vi "Start Sync.vi"(8 "error in (no error)":errorcluster, 11 "gRPC Server in":refnum<class "RouteGuide.lvclass">) -> (0 "error out":errorcluster, 3 "gRPC Server out":refnum<class "RouteGuide.lvclass">)   [LabVIEW 2019, in "route_guide_server.lvlib" / "RouteGuide.lvclass"]
uses:
  RouteGuide.lvclass
  RouteGuide.lvclass/RouteGuide.ctl
  RPC Messages/routeguide_Feature.ctl
  RPC Messages/routeguide_Point.ctl
  RPC Messages/routeguide_RouteSummary.ctl
  Is Call Cancelled Global.vi
  Server Error Global.vi
  route_guide_server.lvlib
  <vilib>/gRPC/LabVIEW gRPC Library/grpc-lvsupport-release.lvlib
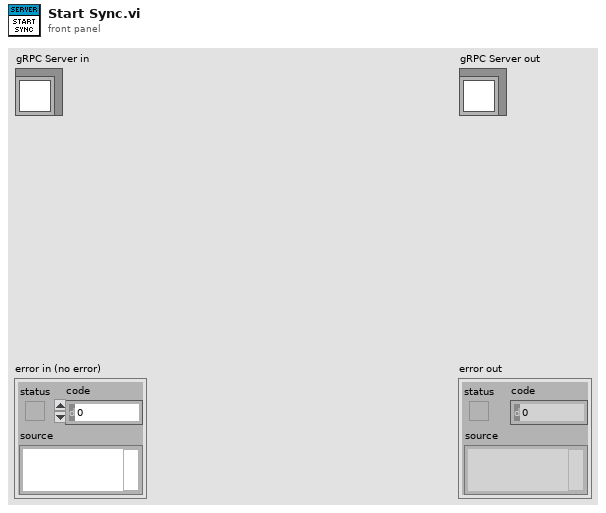
[diagram p1: front panel]
types:
  T1 = typedef "route_guide_server.lvlib/routeguide_Feature.ctl" = cluster{"name":string, "location":T2}
  T2 = typedef "route_guide_server.lvlib/routeguide_Point.ctl" = cluster{"latitude":i32, "longitude":i32}
  T3 = typedef "route_guide_server.lvlib/routeguide_RouteSummary.ctl" = cluster{"point_count":i32, "feature_count":i32, "distance":i32, "elapsed_time":i32}
  T4 = typedef "route_guide_server.lvlib/RouteGuide.lvclass/Server Internal UEs.ctl" = cluster{"routeguide_RouteGuide_GetFeature Internal UE":refnum<user-event>, "routeguide_RouteGuide_ListFeatures Internal UE":refnum<user-event>, "routeguide_RouteGuide_RecordRoute Internal UE":refnum<user-event>, "routeguide_RouteGuide_RouteChat Internal UE":refnum<user-event>}
  T5 = typedef "route_guide_server.lvlib/RouteGuide.lvclass/Server gRPC UEs.ctl" = cluster{"routeguide_RouteGuide_GetFeature gRPC UE":refnum<user-event>, "routeguide_RouteGuide_ListFeatures gRPC UE":refnum<user-event>, "routeguide_RouteGuide_RecordRoute gRPC UE":refnum<user-event>, "routeguide_RouteGuide_RouteChat gRPC UE":refnum<user-event>}
  T6 = typedef "gprc-lvsupport-release.lvlib/grpcId.ctl" = u64
  T7 = typedef "grpc-lvsupport-release.lvlib/grpcId.ctl" = u64
  T8 = typedef "route_guide_server.lvlib/routeguide_Rectangle.ctl" = cluster{"lo":T2, "hi":T2}
  T9 = typedef "route_guide_server.lvlib/routeguide_RouteNote.ctl" = cluster{"location":T2, "message":string}
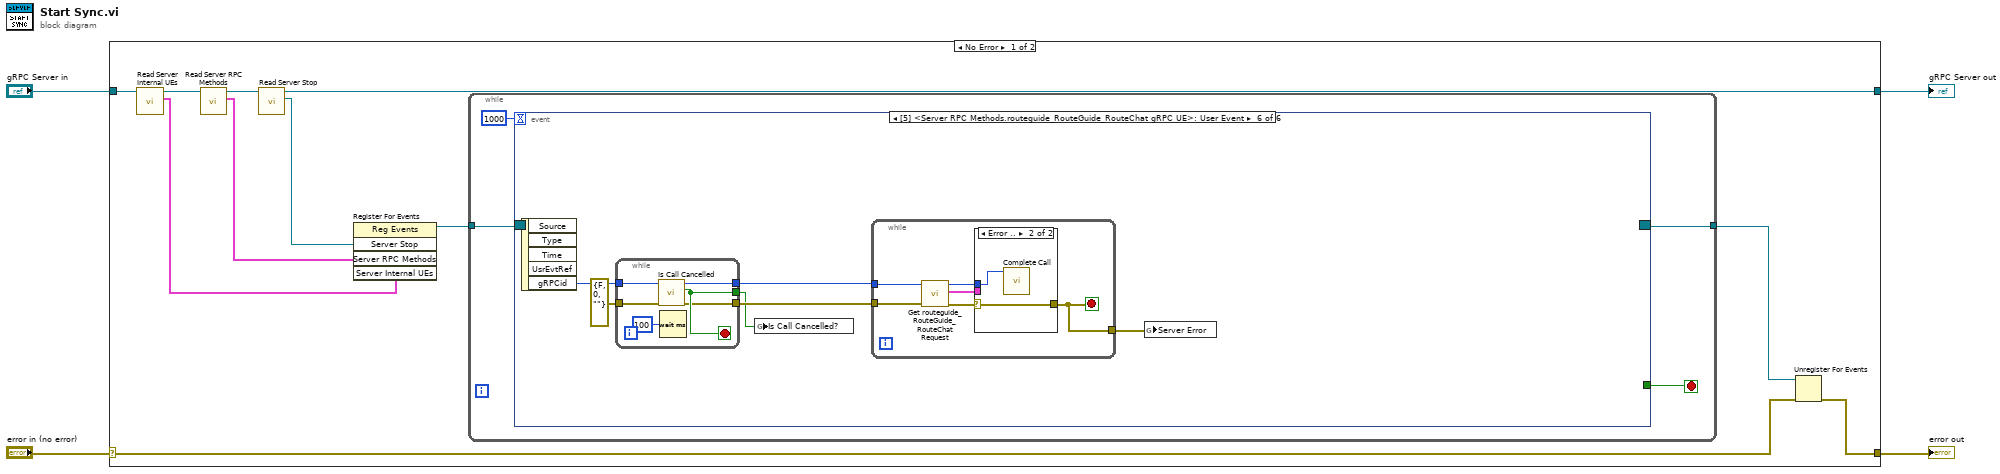
[diagram p0: block diagram]
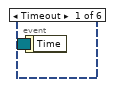
[diagram p2: hidden frame]
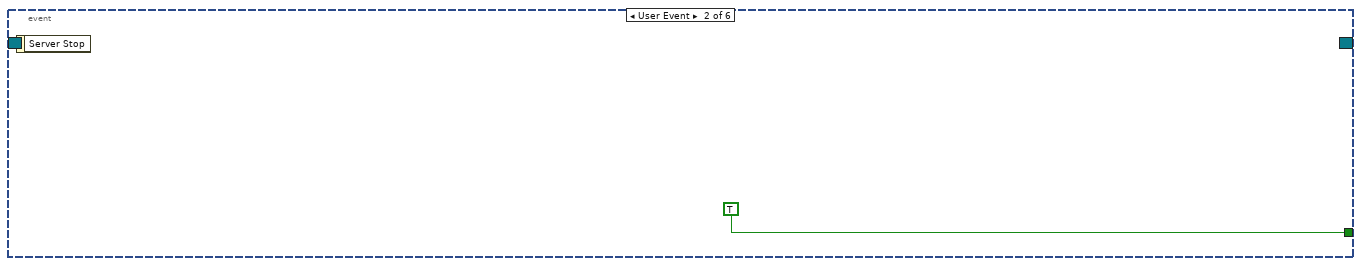
[diagram p3: hidden frame]
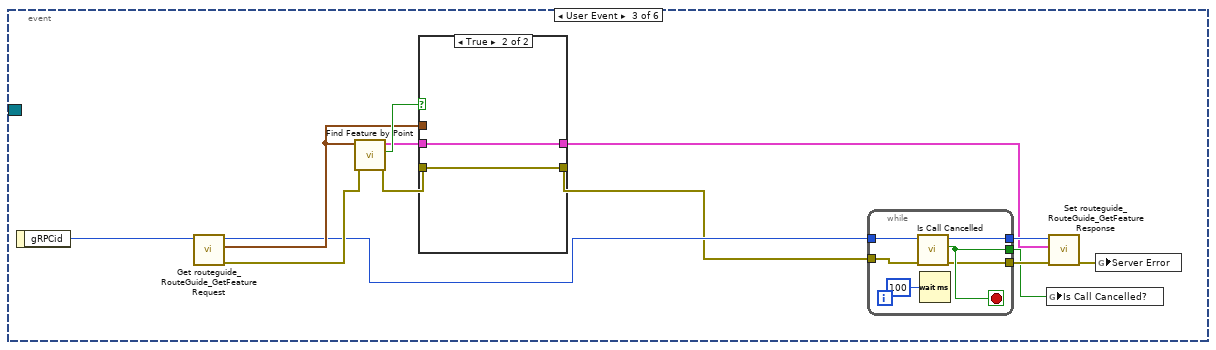
[diagram p4: hidden frame]
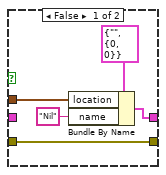
[diagram p5: hidden frame]
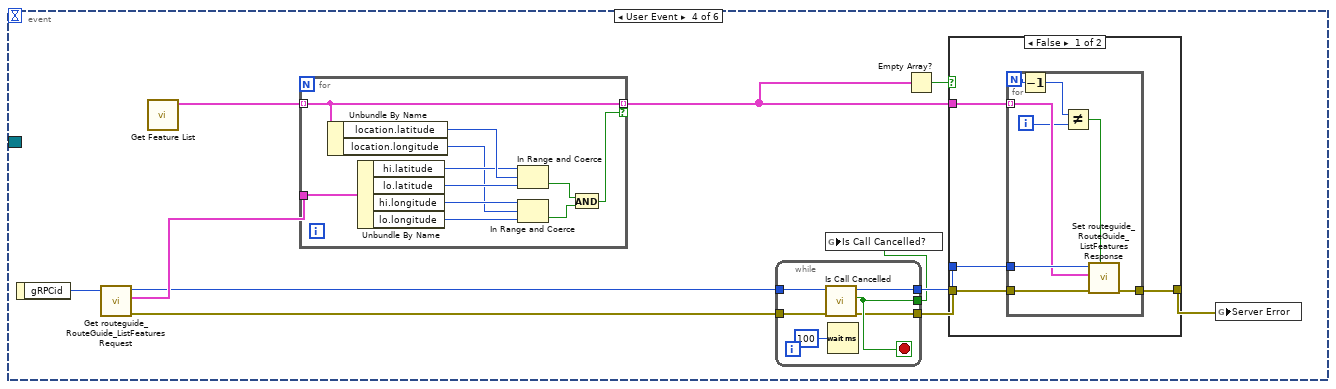
[diagram p6: hidden frame]
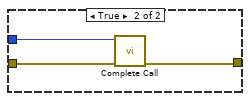
[diagram p7: hidden frame]
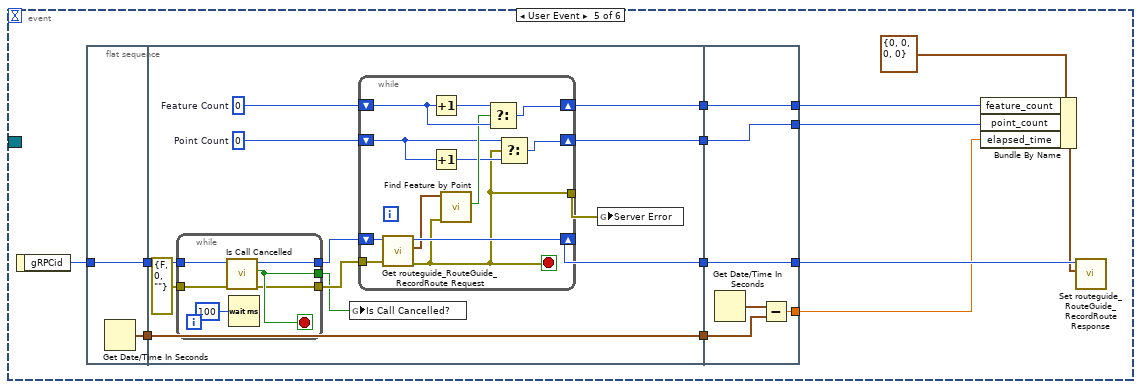
[diagram p8: hidden frame]
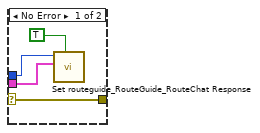
[diagram p9: hidden frame]
diagram:
  n1 = case shown="No Error" "error in (no error)" {
    selector: "error in (no error)" -> [w9 w166]
    tunnel: [w8 w166] -> w3
    tunnel: [w6 w165] -> w1
    tunnel: "gRPC Server in" -> [w15 w165]
    frame No Error {
      n2 = call "Read Server Internal UEs.vi"("SignalGeneratorService in"=w15) -> ("Server Internal UEs"=w13:T4, "SignalGeneratorService out"=w14:refnum<class "RouteGuide.lvclass">)  [unwired: 8 in, 1 out]
      n3 = call "Read Server RPC Methods.vi"("SignalGeneratorService in"=w14) -> ("Server RPC Methods"=w7:T5, "SignalGeneratorService out"=w12:refnum<class "RouteGuide.lvclass">)  [unwired: 8 in, 1 out]
      n4 = call-dynamic "Read Server Stop.vi"("iService in"=w12) -> ("Server Stop"=w5:refnum<user-event>, "iService out"=w6:refnum<class "RouteGuide.lvclass">)  [unwired: 8 in, 1 out]
      n5 = register-events(w5, w7, w13) -> (reference out=w11:refnum<event-registration>)  [unwired: 2 in, 1 out]
      n6 = while {
        tunnel: w11 -> [w19]
        tunnel: [w17] -> w10
        stop <- w18 stop-if-true
        n7 = event "RPC Methods Event Structure" shown="[5] <Server RPC Methods.routeguide_RouteGuide_RouteChat gRPC UE>: User Event" {
          selector: w19 -> [_ _ _ _ _ _]
          dyn-events: [_ _ _ _ _ _] -> w17
          timeout: 1000 -> [_ _ _ _ _ _]
          tunnel: [_ TRUE _ _ _ _] -> w18
          event Timeout {
            n8 = event-data() -> ()  [unwired: 1 in, 1 out]
          }
          event User Event {
            n9 = event-data() -> ()  [unwired: 1 in, 1 out]
          }
          event User Event {
            n10 = event-data() -> ("gRPCid"=w33:T6)  [unwired: 1 in]
            n11 = call "Get routeguide_RouteGuide_GetFeature Request.vi"("gRPCid in"=w33) -> ("error out"=w32:errorcluster, "Message Data"=w28:T2, "gRPCid out"=w27:T7)  [unwired: 8 in]
            n12 = call "Find Feature by Point.vi"("error in"=w32, "Point"=w28) -> ("error out"=w29:errorcluster, "Found?"=w31:bool, "Feature"=w30:cluster{"name":string, "location":T2})  [unwired: 7 in]
            n13 = case shown="True" w31 {
              tunnel: w30 -> [_ w46]
              tunnel: w29 -> [w44 w45]
              tunnel: [w42 w46] -> w24
              tunnel: [w44 w45] -> w26
              tunnel: w28 -> [w41 _]
              frame False {
                n14 = Bundle By Name(cluster=T1 {"name"="", "location"={"latitude"=0, "longitude"=0}} ("Message Data"), "location"=w41, "name"="Nil") -> (w42:T1)
              }
              frame True {
              }
            }
            n15 = while {
              tunnel: w27 -> [w39]
              tunnel: w26 -> [w38]
              tunnel: [w37] -> w21
              tunnel: [w36] -> w25
              tunnel: [w35] -> w23
              stop <- w37 stop-if-true
              n16 = call <vilib>:"Is Call Cancelled.vi"("error in"=w38, "gRPCid in"=w39) -> ("error out"=w35:errorcluster, "Is Cancelled"=w37:bool, "gRPCid out"=w36:T7)  [unwired: 7 in]
              n17 = Wait (ms)(milliseconds to wait=u32 100) -> ()  [unwired: 1 out]
            }
            n18 = global write "Is Call Cancelled Global.vi" "Is Call Cancelled?"(w21) -> ()
            n19 = call "Set routeguide_RouteGuide_GetFeature Response.vi"("error in (no error)"=w23, "Message Data"=w24, "gRPCid in"=w25) -> ("error out"=w22:errorcluster)  [unwired: 8 in]
            n20 = global write "Server Error Global.vi" "Server Error"(w22) -> ()
          }
          event User Event {
            n21 = event-data() -> ("gRPCid"=w57:T6)  [unwired: 1 in]
            n22 = call "Get routeguide_RouteGuide_ListFeatures Request.vi"("gRPCid in"=w57) -> ("error out"=w49:errorcluster, "Message Data"=w55:T8, "gRPCid out"=w51:T7)  [unwired: 8 in]
            n23 = call "Get Feature List.vi"() -> ("Feature List"=w56:cluster{"name":string, "location":T2}[])  [unwired: 10 in, 1 out]
            n24 = for {
              tunnel: w56 -> [w80] mode=indexing
              tunnel: w55 -> [w89]
              tunnel: [w80] -> w53 mode=indexing if=w79
              n25 = Unbundle By Name(w80) -> ("location.latitude"=w88:i32, "location.longitude"=w83:i32)
              n26 = Unbundle By Name(w89) -> ("hi.latitude"=w87:i32, "lo.latitude"=w86:i32, "hi.longitude"=w85:i32, "lo.longitude"=w84:i32)
              n27 = In Range and Coerce(upper limit=w87, x=w88, lower limit=w86) -> (In Range?=w81:bool)  [unwired: 1 out]
              n28 = In Range and Coerce(upper limit=w85, x=w83, lower limit=w84) -> (In Range?=w82:bool)  [unwired: 1 out]
              n29 = And(x=w81, y=w82) -> (x .and. y?=w79:bool)
            }
            n30 = while {
              tunnel: w51 -> [w63]
              tunnel: w49 -> [w62]
              tunnel: [w61] -> w47
              tunnel: [w60] -> w50
              tunnel: [w59] -> w48
              stop <- w61 stop-if-true
              n31 = call <vilib>:"Is Call Cancelled.vi"("error in"=w62, "gRPCid in"=w63) -> ("error out"=w59:errorcluster, "Is Cancelled"=w61:bool, "gRPCid out"=w60:T7)  [unwired: 7 in]
              n32 = Wait (ms)(milliseconds to wait=u32 100) -> ()  [unwired: 1 out]
            }
            n33 = global write "Is Call Cancelled Global.vi" "Is Call Cancelled?"(w47) -> ()
            n34 = Empty Array?(array=w53) -> (empty?=w54:bool)
            n35 = case shown="False" w54 {
              tunnel: w50 -> [w67 w77]
              tunnel: w48 -> [w66 w78]
              tunnel: w53 -> [w65 _]
              tunnel: [w64 w76] -> w52
              frame False {
                n36 = for {
                  N -> [w72]
                  tunnel: w67 -> [w75]
                  tunnel: w66 -> [w74]
                  tunnel: w65 -> [w73] mode=indexing
                  tunnel: [w68] -> w64
                  i -> [w71]
                  n37 = Decrement(x=w72) -> (x-1=w70:i32)
                  n38 = Not Equal?(x=w70, y=w71) -> (x != y?=w69:bool)
                  n39 = call "Set routeguide_RouteGuide_ListFeatures Response.vi"("Streeming? (F)"=w69, "error in (no error)"=w74, "Message Data"=w73, "gRPCid in"=w75) -> ("error out"=w68:errorcluster)  [unwired: 7 in]
                }
              }
              frame True {
                n40 = call <vilib>:"Complete Call.vi"("gRPCid"=w77, "error in"=w78) -> ("error out"=w76:errorcluster)  [unwired: 8 in]
              }
            }
            n41 = global write "Server Error Global.vi" "Server Error"(w52) -> ()
          }
          event User Event {
            n42 = event-data() -> ("gRPCid"=w102:T6)  [unwired: 1 in]
            n43 = flat-sequence {
              tunnel: w102 -> [w104]
              tunnel: [w104] -> w97
              tunnel: [w103] -> w92
              tunnel: w97 -> [w109]
              tunnel: [w116] -> w96
              tunnel: [w111] -> w95
              tunnel: [w114] -> w94
              tunnel: w92 -> [w113]
              tunnel: [w113] -> w91
              tunnel: [w139] -> w99
              tunnel: [w140] -> w101
              tunnel: w96 -> [w140]
              tunnel: w95 -> [w139]
              tunnel: [w138] -> w93
              tunnel: w94 -> [w138]
              tunnel: w91 -> [w136]
              tunnel: [w135] -> w90
              frame #0 {
                n44 = Get Date/Time In Seconds() -> (seconds since 1Jan1904=w103:timestamp)
              }
              frame #1 {
                w112 = 0  # Point Count
                w115 = 0  # Feature Count
                n45 = while {
                  tunnel: w109 -> [w122]
                  tunnel: errorcluster {"status"=FALSE, "code"=0, "source"=""} ("error out") -> [w121]
                  tunnel: [w120] -> w105
                  tunnel: [w119] -> w107
                  tunnel: [w118] -> w106
                  stop <- w120 stop-if-true
                  n46 = call <vilib>:"Is Call Cancelled.vi"("error in"=w121, "gRPCid in"=w122) -> ("error out"=w118:errorcluster, "Is Cancelled"=w120:bool, "gRPCid out"=w119:T7)  [unwired: 7 in]
                  n47 = Wait (ms)(milliseconds to wait=u32 100) -> ()  [unwired: 1 out]
                }
                n48 = global write "Is Call Cancelled Global.vi" "Is Call Cancelled?"(w105) -> ()
                n49 = while {
                  shift-right: [w133] -> w116
                  shift-left: w107 -> [w134]
                  shift-right: [w131] -> w114
                  shift-left: w115 -> [w130]
                  shift-right: [w127] -> w111
                  shift-left: w112 -> [w125]
                  tunnel: [w124] -> w110
                  tunnel: w106 -> [w123]
                  stop <- w124 stop-if-true
                  n50 = call "Get routeguide_RouteGuide_RecordRoute Request.vi"("error in (no error)"=w123, "gRPCid in"=w134) -> ("error out"=w124:errorcluster, "Message Data"=w132:T2, "gRPCid out"=w133:T7)  [unwired: 7 in]
                  n51 = Increment(x=w130) -> (x+1=w129:i32)
                  n52 = Increment(x=w125) -> (x+1=w126:i32)
                  n53 = call "Find Feature by Point.vi"("error in"=w124, "Point"=w132) -> ("Found?"=w128:bool)  [unwired: 7 in, 2 out]
                  n54 = Select(t=w129, s=w128, f=w130) -> (s? t:f=w131:i32)
                  n55 = Select(t=w125, s=w124, f=w126) -> (s? t:f=w127:i32)
                }
                n56 = global write "Server Error Global.vi" "Server Error"(w110) -> ()
              }
              frame #2 {
                n57 = Get Date/Time In Seconds() -> (seconds since 1Jan1904=w137:timestamp)
                n58 = Subtract(x=w137, y=w136) -> (x-y=w135:dbl)
              }
            }
            n59 = Bundle By Name(cluster=T3 {"point_count"=0, "feature_count"=0, "distance"=0, "elapsed_time"=0} ("Message Data"), "feature_count"=w93, "point_count"=w99, "elapsed_time"=w90) -> (w98:T3)
            n60 = call "Set routeguide_RouteGuide_RecordRoute Response.vi"("Message Data"=w98, "gRPCid in"=w101) -> ()  [unwired: 9 in, 1 out]
          }
          event User Event {
            n61 = event-data() -> ("gRPCid"=w145:T6)  [unwired: 1 in, 4 out]
            n62 = while {
              tunnel: w145 -> [w152]
              tunnel: errorcluster {"status"=FALSE, "code"=0, "source"=""} ("error out") -> [w151]
              tunnel: [w150] -> w141
              tunnel: [w149] -> w144
              tunnel: [w148] -> w142
              stop <- w150 stop-if-true
              n63 = call <vilib>:"Is Call Cancelled.vi"("error in"=w151, "gRPCid in"=w152) -> ("error out"=w148:errorcluster, "Is Cancelled"=w150:bool, "gRPCid out"=w149:T7)  [unwired: 7 in]
              n64 = Wait (ms)(milliseconds to wait=u32 100) -> ()  [unwired: 1 out]
            }
            n65 = global write "Is Call Cancelled Global.vi" "Is Call Cancelled?"(w141) -> ()
            n66 = while {
              tunnel: w144 -> [w158]
              tunnel: [w154] -> w146
              tunnel: w142 -> [w153]
              stop <- w154 stop-if-true
              n67 = call "Get routeguide_RouteGuide_RouteChat Request.vi"("error in (no error)"=w153, "gRPCid in"=w158) -> ("error out"=w155:errorcluster, "Message Data"=w156:T9, "gRPCid out"=w157:T7)  [unwired: 7 in]
              n68 = case shown="Error .." w155 {
                selector: w155 -> [w160 w164]
                tunnel: w157 -> [w162 w163]
                tunnel: w156 -> [w161 _]
                tunnel: [w160 w164] -> w154
                frame No Error {
                  n69 = call "Set routeguide_RouteGuide_RouteChat Response.vi"("Streeming? (F)"=TRUE, "Message Data"=w161, "gRPCid in"=w162) -> ()  [unwired: 8 in, 1 out]
                }
                frame Error {
                  n70 = call <vilib>:"Complete Call.vi"("gRPCid"=w163) -> ()  [unwired: 9 in, 1 out]
                }
              }
            }
            n71 = global write "Server Error Global.vi" "Server Error"(w146) -> ()
          }
        }
      }
      n72 = Unregister For Events(event registration refnum=w10, error in=w9) -> (error out=w8:errorcluster)
    }
    frame Error {
    }
  }
  "error out" <- w3
  "gRPC Server out" <- w1
